vi "Auto Scorer.vi"() -> ()   [LabVIEW 2024, in "Wordle Scorer.lvlib"]
uses:
  Wordle Scorer.lvlib
  Scorer State.ctl
  Scoring Result.ctl
panel:
  out "tskill output":string
  in  "Poll Now":bool
  out "Response":string
  out "Scoring Result":T1
  out "Run Time":dbl format="%<%M:%S%1u>t"
  out "Run Start":timestamp
  out "VI Refnum":refnum<vi>
  out "App Ref":refnum<vi>
  out "Zip":path
  out "Upload Error":errorcluster
  out "Score Error":errorcluster
  out "Download Error":errorcluster
  out "Poll Error":errorcluster
  out "Last Poll":timestamp format="%<%Y-%m-%d %H:%M:%S>T"
  out "State":T2
  out "Previous Submission":i32
  out "Current Submission":i32
  out "Time to next poll":dbl format="%#.0f"
  in  "Poll Period":dbl=60.0
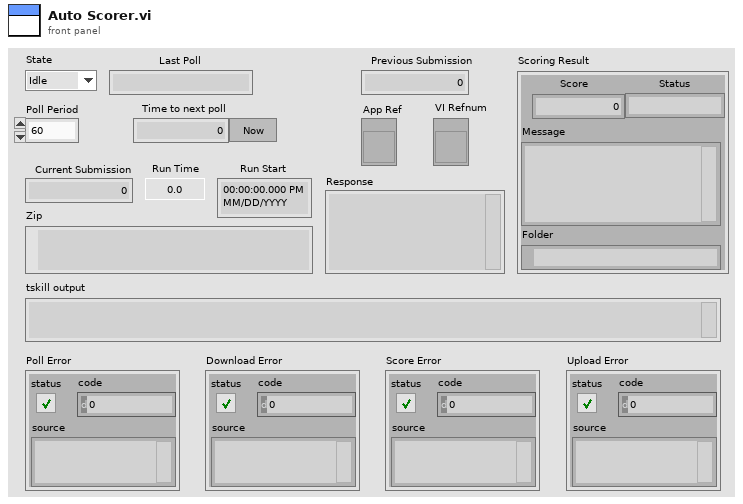
[diagram p1: front panel]
types:
  T1 = typedef "Wordle Scorer.lvlib/Scoring Result.ctl" = cluster{"Score":dbl, "Status":string, "Message":string, "Folder":path}
  T2 = typedef "Wordle Scorer.lvlib/Scorer State.ctl" = enum16{"Idle", "Poll", "Run", "Upload", "Error", "Timeout"}
  T3 = enum32{"Bad", "Idle", "Run top level", "Running"}
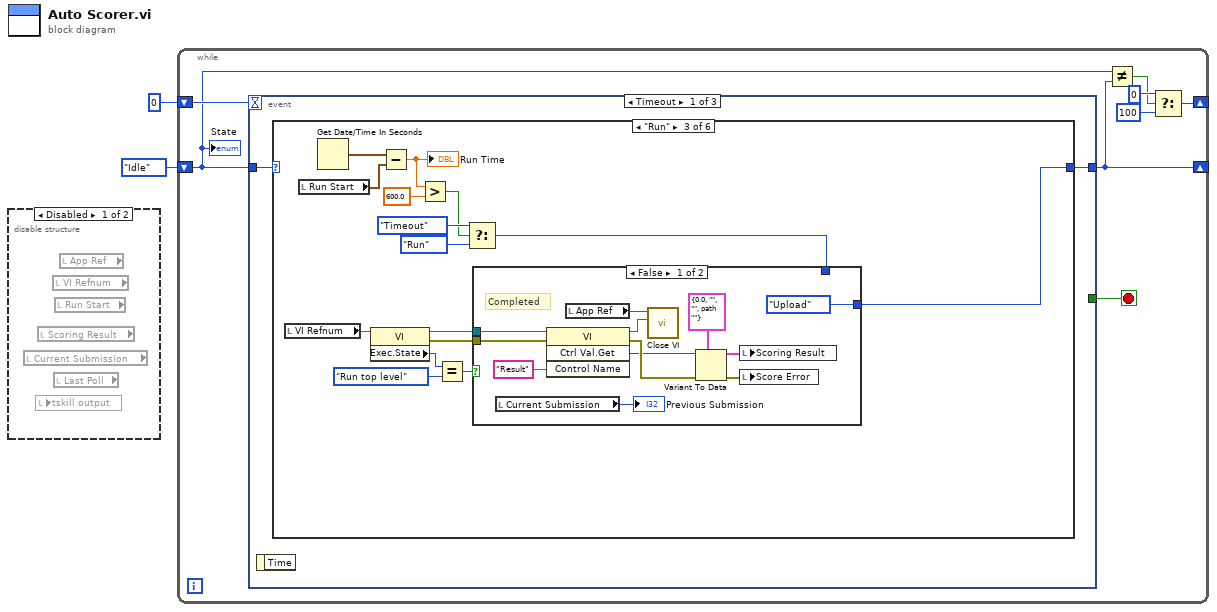
[diagram p0: block diagram]
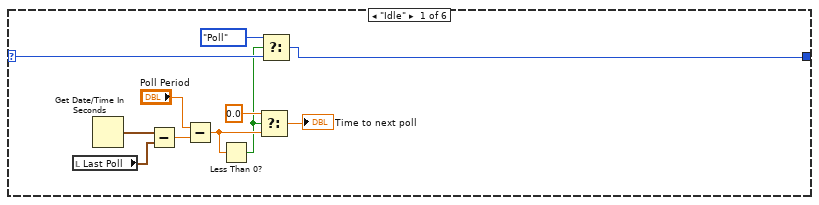
[diagram p3: hidden frame]
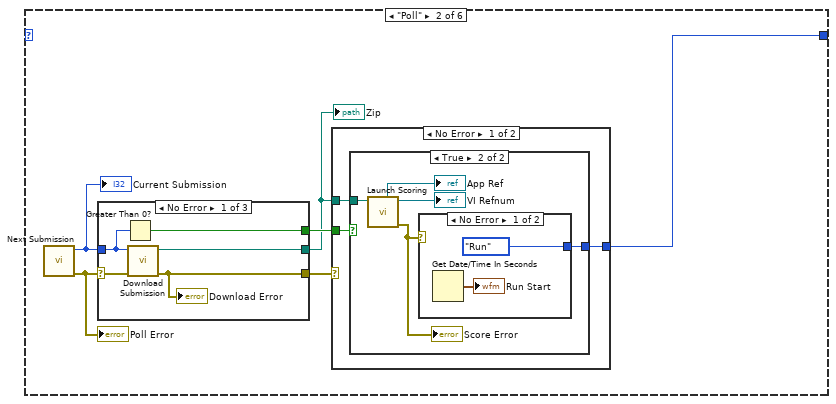
[diagram p4: hidden frame]
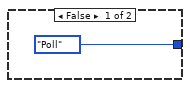
[diagram p5: hidden frame]
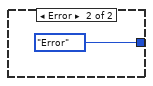
[diagram p6: hidden frame]
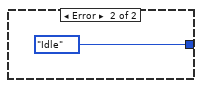
[diagram p7: hidden frame]
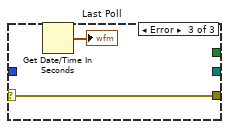
[diagram p9: hidden frame]
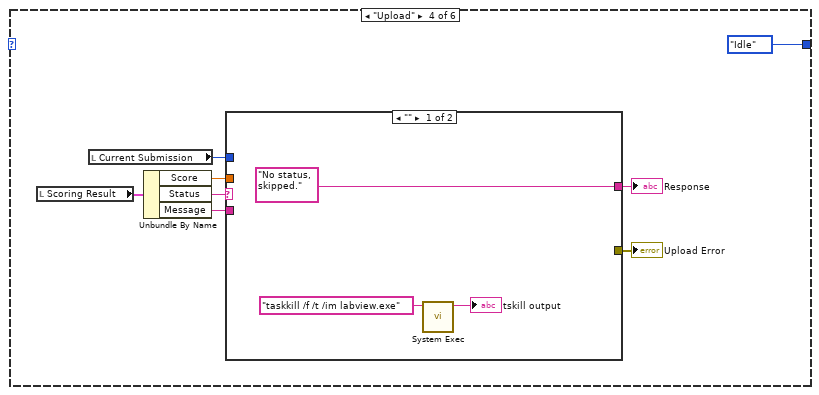
[diagram p11: hidden frame]
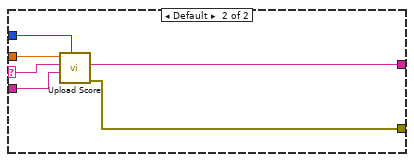
[diagram p12: hidden frame]
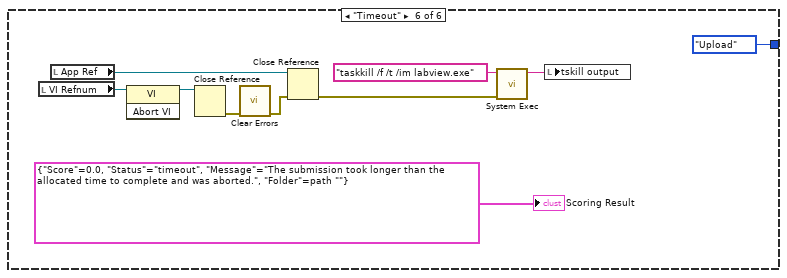
[diagram p14: hidden frame]
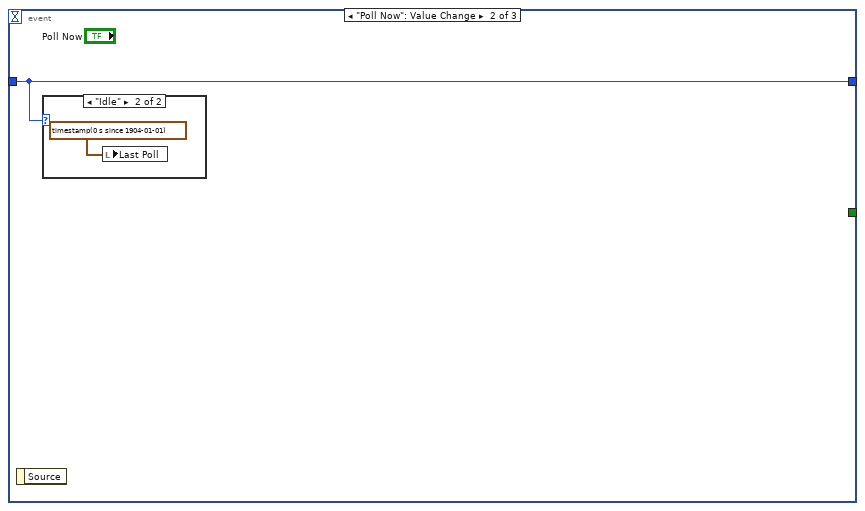
[diagram p15: hidden frame]
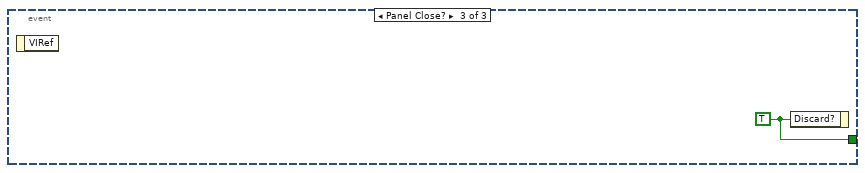
[diagram p17: hidden frame]
diagram:
  n1 = disable-structure shown="Disabled" {
    frame Disabled {
      n2 = local read "Current Submission"() -> ()  [unwired: 1 out]
      n3 = local read "tskill output"() -> ()  [unwired: 1 in]
      n4 = local read "Scoring Result"() -> ()  [unwired: 1 out]
      n5 = local read "VI Refnum"() -> ()  [unwired: 1 out]
      n6 = local read "Last Poll"() -> ()  [unwired: 1 out]
      n7 = local read "Run Start"() -> ()  [unwired: 1 out]
      n8 = local read "App Ref"() -> ()  [unwired: 1 out]
    }
    frame Enabled {
    }
  }
  n9 = while {
    shift-right: [w9] -> _
    shift-left: Scorer_State."Idle" ("Scorer State") -> [w8]
    shift-right: [w6] -> _
    shift-left: 0 -> [w10]
    stop <- w3 stop-if-true
    n10 = event shown="[0] Timeout" {
      selector: _ -> [_ _ _]
      dyn-events: _ -> [_ _ _]
      timeout: w10 -> [_ _ _]
      tunnel: w8 -> [w12 w107 _]
      tunnel: [w11 w107 _] -> w9
      tunnel: [_ _ w109] -> w3
      event Timeout {
        n11 = event-data() -> ()  [unwired: 1 in, 1 out]
        n12 = case shown="\"Run\"" w12 {
          selector: w12 -> [w16 _ _ _ w96 _]
          tunnel: [w13 w26 w59 Scorer_State."Idle" ("Scorer State") w96 Scorer_State."Upload" ("Scorer State")] -> w11
          frame "Idle" {
            n13 = local read "Last Poll"() -> (w22:timestamp)
            n14 = Get Date/Time In Seconds() -> (seconds since 1Jan1904=w23:timestamp)
            n15 = Subtract(x=w23, y=w22) -> (x-y=w21:dbl)
            n16 = Subtract(x="Poll Period", y=w21) -> (x-y=w19:dbl)
            n17 = Less Than 0?(x=w19) -> (x < 0?=w15:bool)
            n18 = Select(t=0.0, s=w15, f=w19) -> (s? t:f=→"Time to next poll":dbl)
            n19 = Select(t=Scorer_State."Poll", s=w15, f=w16) -> (s? t:f=w13:T2)
          }
          frame "Poll" {
            n20 = call "Next Submission.vi"() -> ("error out"=w28:errorcluster, "submission"=w24:i32)  [unwired: 9 in, 1 out]
            "Poll Error" <- w28
            "Current Submission" <- w24
            n21 = case shown="No Error" w28 {
              selector: w28 -> [w46 w48 w49]
              tunnel: w24 -> [w47 _ _]
              tunnel: [w45 _ _] -> w25
              tunnel: [w44 w48 w49] -> w29
              tunnel: [w43 _ _] -> w27
              frame No Error {
                n22 = Greater Than 0?(x=w47) -> (x > 0?=w43:bool)
                n23 = call "Download Submission.vi"("error in (no error)"=w46, "submission"=w47) -> ("error out"=w44:errorcluster, "Zip Path"=w45:path)  [unwired: 7 in, 1 out]
                "Download Error" <- w44
              }
              frame Default {
              }
              frame Error {
                # "No submissions"
                n24 = Get Date/Time In Seconds() -> (seconds since 1Jan1904=→"Last Poll":timestamp)
              }
            }
            "Zip" <- w25
            n25 = case shown="No Error" w29 {
              tunnel: w27 -> [w32 _]
              tunnel: [w31 Scorer_State."Idle" ("Scorer State")] -> w26
              tunnel: w25 -> [w30 _]
              frame No Error {
                n26 = case shown="True" w32 {
                  tunnel: [Scorer_State."Poll" ("Scorer State") w37] -> w31
                  tunnel: w30 -> [_ w34]
                  frame False {
                  }
                  frame True {
                    n27 = call "Launch Scoring.vi"("Zip"=w34) -> ("error out"=w38:errorcluster, "VI Refnum"=→"VI Refnum":refnum<vi>, "App Ref"=→"App Ref":refnum<vi>)  [unwired: 8 in]
                    "Score Error" <- w38
                    n28 = case shown="No Error" w38 {
                      tunnel: [Scorer_State."Run" ("Scorer State") Scorer_State."Error" ("Scorer State")] -> w37
                      frame No Error {
                        n29 = Get Date/Time In Seconds() -> (seconds since 1Jan1904=→"Run Start":timestamp)
                      }
                      frame Error {
                      }
                    }
                  }
                }
              }
              frame Error {
              }
            }
          }
          frame "Run" {
            n30 = local read "VI Refnum"() -> (w65:refnum<vi>)
            n31 = local read "Run Start"() -> (w61:timestamp)
            n32 = Get Date/Time In Seconds() -> (seconds since 1Jan1904=w62:timestamp)
            n33 = property class="VI"(reference=w65) -> (reference out=w52:refnum<vi>, error out=w51:errorcluster, "Exec.State"=w64:T3)  [unwired: 1 in]
            n34 = Subtract(x=w62, y=w61) -> (x-y=w58:dbl)
            "Run Time" <- w58
            n35 = Greater?(x=w58, y=600.0) -> (0:w54:bool)
            n36 = Equal?(x=w64, y=T3."Run top level") -> (x = y?=w60:bool)
            n37 = Select(t=Scorer_State."Timeout" ("Scorer State"), s=w54, f=Scorer_State."Run" ("Scorer State")) -> (s? t:f=w53:T2)
            n38 = case shown="False" w60 {
              tunnel: [Scorer_State."Upload" ("Scorer State") w78] -> w59
              tunnel: w53 -> [_ w78]
              tunnel: w52 -> [w76 _]
              tunnel: w51 -> [w73 _]
              frame False {
                # "Completed"
                n39 = local read "Current Submission"() -> (→"Previous Submission":i32)
                n40 = invoke class="VI" method="Ctrl Val.Get"(reference=w76, error in=w73, "Control Name"="Result") -> (reference out=w67:refnum<vi>, error out=w77:errorcluster, "Get Control Value Variant"=w74:variant)  [unwired: 1 in, 1 out]
                n41 = local read "App Ref"() -> (w66:refnum<vi>)
                n42 = call "Close VI.vi"("VI Refnum"=w67, "App Ref"=w66) -> ()  [unwired: 10 in]
                n43 = Variant To Data(error in=w77, type=T1 {"Score"=0.0, "Status"="", "Message"="", "Folder"=path ""} ("Scoring Result"), Variant=w74) -> (data=w71:T1, error out=w70:errorcluster)
                n44 = local write "Scoring Result"(w71) -> ()
                n45 = local write "Score Error"(w70) -> ()
              }
              frame True {
                # "Still running"
              }
            }
          }
          frame "Upload" {
            n46 = local read "Scoring Result"() -> (w85:T1)
            n47 = local read "Current Submission"() -> (w83:i32)
            n48 = Unbundle By Name(w85) -> ("Score"=w84:dbl, "Status"=w82:string, "Message"=w81:string)
            n49 = case shown="\"\"" w82 {
              selector: w82 -> [_ w93]
              tunnel: w84 -> [_ w95]
              tunnel: w83 -> [_ w94]
              tunnel: w81 -> [_ w92]
              tunnel: [_ w91] -> w80
              tunnel: ["No status, skipped." ("Response") w90] -> w79
              frame "" {
                n50 = call <vilib>:"System Exec.vi"("command line"="taskkill /f /t /im labview.exe") -> ("standard output"=→"tskill output":string)  [unwired: 7 in, 3 out]
              }
              frame Default {
                n51 = call "Upload Score.vi"("submission"=w94, "result"=w92, "status"=w93, "Run Time"=w95) -> ("error out"=w91:errorcluster, "Response"=w90:string)  [unwired: 5 in, 1 out]
              }
            }
            "Upload Error" <- w80
            "Response" <- w79
          }
          frame "Error" {
            # "Whoops! Time to be saved!"
          }
          frame "Timeout" {
            n52 = local read "VI Refnum"() -> (w104:refnum<vi>)
            n53 = local read "App Ref"() -> (w100:refnum<vi>)
            n54 = invoke class="VI" method="Abort VI"(reference=w104) -> (reference out=w103:refnum<vi>)  [unwired: 2 in, 2 out]
            n55 = Close Reference(reference=w103) -> (error out=w102:errorcluster)  [unwired: 1 in]
            n56 = call <vilib>:"Clear Errors.vi"("error in (no error)"=w102) -> ("error out"=w101:errorcluster)  [unwired: 5 in, 1 out]
            n57 = Close Reference(reference=w100, error in (no error)=w101) -> (error out=w98:errorcluster)
            n58 = call <vilib>:"System Exec.vi"("error in (no error)"=w98, "command line"="taskkill /f /t /im labview.exe") -> ("standard output"=w97:string)  [unwired: 6 in, 3 out]
            n59 = local write "tskill output"(w97) -> ()
            "Scoring Result" <- T1 {"Score"=0.0, "Status"="timeout", "Message"="The submission took longer than the allocated time to complete and was aborted.", "Folder"=path ""} ("Scoring Result")
          }
        }
      }
      event "Poll Now": Value Change {
        n60 = event-data() -> ()  [unwired: 1 in, 1 out]
        n61 = case shown="\"Idle\"" w107 {
          frame Default {
          }
          frame "Idle" {
            n62 = local write "Last Poll"(timestamp(0 s since 1904-01-01) ("Last Poll")) -> ()
          }
        }
      }
      event Panel Close? {
        w109 = TRUE ("Discard?")
        n63 = event-data() -> ()  [unwired: 1 in, 1 out]
        n64 = event-data("Discard?"=w109) -> ()  [unwired: 1 in, 1 out]
      }
    }
    n65 = Not Equal?(x=w8, y=w9) -> (x != y?=w4:bool)
    n66 = Select(t=0, s=w4, f=100) -> (s? t:f=w6:i32)
    "State" <- w8
  }
